vi "Test ISO8601 Conversions.vi"(8 "error in (no error)":errorcluster) -> (0 "error out":errorcluster)   [LabVIEW 2013]
uses:
  source/Timestamp Compare Units -- enum.ctl
  source/formatter.iso8601/ISO8601 Date Formats.ctl
  <vilib>/addons/_JKI Toolkits/Caraya/classes/Assert/Assert True.vi
  source/EpochNotTimestamp.vi
  <vilib>/addons/_JKI Toolkits/Caraya/classes/Assert/Assert.lvclass
  <vilib>/addons/_JKI Toolkits/Caraya/classes/Test/Test.lvclass
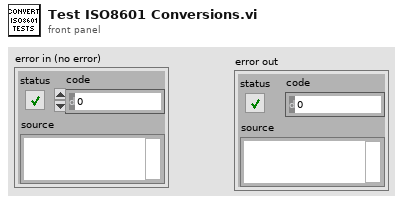
[diagram p1: front panel]
types:
  T1 = typedef "ISO8601 Date Formats.ctl" = enum16{"UTC Date-Time", "ISO Time", "Date", "Calendar Month", "Week", "Week-Day", "Month-Day", "Ordinal Date"}
  T2 = typedef "Timestamp Compare Units -- enum.ctl" = enum16{"week", "day", "hour", "minute", "second", "millisecond", "microsecond", "nanosecond"}
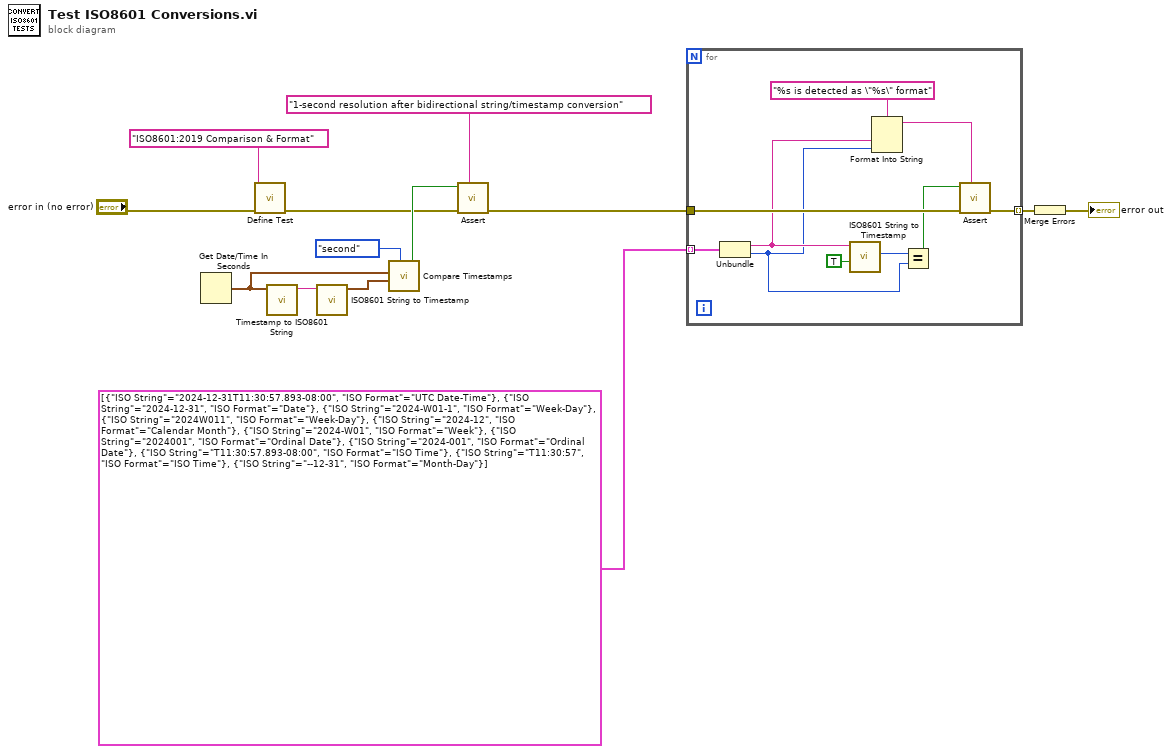
[diagram p0: block diagram]
diagram:
  n1 = Get Date/Time In Seconds() -> (seconds since 1Jan1904=w6:timestamp)
  n2 = call <vilib>:"Define Test.vi"("error in (no error)"="error in (no error)", "Label (VI Title)"="ISO8601:2019 Comparison & Format") -> ("error out"=w7:errorcluster)  [unwired: 8 in, 1 out]
  n3 = call "Timestamp to ISO8601 String.vi"("Timestamp (now)"=w6) -> ("ISO8601 String"=w5:string)  [unwired: 10 in]
  n4 = call "ISO8601 String to Timestamp.vi"("ISO8601 String"=w5) -> ("Timestamp"=w10:timestamp)  [unwired: 8 in, 2 out]
  n5 = call "Compare Timestamps.vi"("Unit (ms)"=Timestamp_Compare_Units_--_enum."second", "timestamp (1)"=w6, "timestamp (2)"=w10) -> ("Equal?"=w11:bool)  [unwired: 5 in]
  n6 = call-poly <vilib>:"Assert.vi"("Label"="1-second resolution after bidirectional string/timestamp conversion" ("x"), "error in (no error)"=w7, "True?"=w11) -> ("error out"=w4:errorcluster)  [unwired: 7 in, 1 out]
  n7 = for {
    tunnel: w4 -> [w21]
    tunnel: [w20] -> w3 mode=indexing
    tunnel: cluster{"ISO String":string, "ISO Format":T1}[] [{"ISO String"="2024-12-31T11:30:57.893-08:00", "ISO Format"=enum."UTC Date-Time"}, {"ISO String"="2024-12-31", "ISO Format"=enum."Date"}, {"ISO String"="2024-W01-1", "ISO Format"=enum."Week-Day"}, {"ISO String"="2024W011", "ISO Format"=enum."Week-Day"}, {"ISO String"="2024-12", "ISO Format"=enum."Calendar Month"}, {"ISO String"="2024-W01", "ISO Format"=enum."Week"}, {"ISO String"="2024001", "ISO Format"=enum."Ordinal Date"}, {"ISO String"="2024-001", "ISO Format"=enum."Ordinal Date"}, {"ISO String"="T11:30:57.893-08:00", "ISO Format"=enum."ISO Time"}, {"ISO String"="T11:30:57", "ISO Format"=enum."ISO Time"}, {"ISO String"="--12-31", "ISO Format"=enum."Month-Day"}] -> [w14] mode=indexing
    n8 = Unbundle(w14) -> ("ISO String"=w17:string, "ISO Format"=w15:T1)
    n9 = call "ISO8601 String to Timestamp.vi"("Strict ISO? (T)"=TRUE, "ISO8601 String"=w17) -> ("ISO Format"=w22:T1)  [unwired: 7 in, 2 out]
    n10 = Format Into String(format string="%s is detected as \"%s\" format", w17, w15) -> (resulting string=w18:string)  [unwired: 2 in, 1 out]
    n11 = Equal?(x=w22, y=w15) -> (x = y?=w19:bool)
    n12 = call-poly <vilib>:"Assert.vi"("Label"=w18, "error in (no error)"=w21, "True?"=w19) -> ("error out"=w20:errorcluster)  [unwired: 7 in, 1 out]
  }
  n13 = Merge Errors(w3) -> (→"error out":errorcluster)
